vi "get device name.vi"(8 "error in (no error)":errorcluster, 10 "device_index":i32, 11 "device_enumeration":u32) -> (0 "error out":errorcluster, 3 "function return":string)   [LabVIEW 2020, in "libximc.lvlib"]
doc: "pchar XIMC_API get_device_name(device_enumeration_t device_enumeration, int device_index);"
uses:
  libximc.lvlib
  libximc.dll
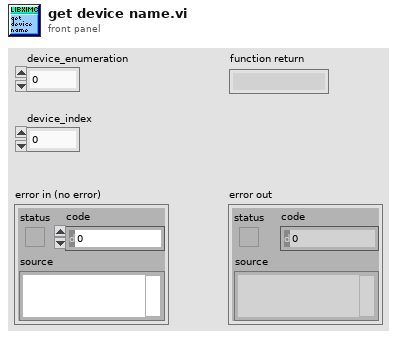
[diagram p1: front panel]
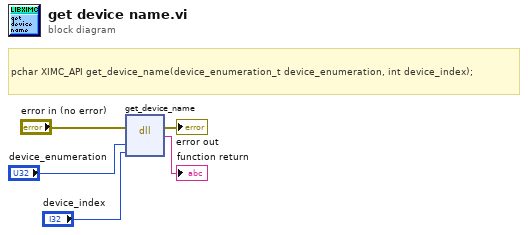
[diagram p0: block diagram]
diagram:
  # "pchar XIMC_API get_device_name(device_enumeration_t device_enumeration, int device_index);"
  n1 = dll-call lib="E:/Norway Project/All Hardware/New Microscope/LabVIEW/Stage/libximc.*" fn="get_device_name"(error in="error in (no error)", "device_enumeration"="device_enumeration", "device_index"="device_index") -> (error out=→"error out":errorcluster, →"function return":string)  [unwired: 4 in, 1 out]
